vi "potentialField.vi"(5 "Ball":refnum<class "Ball.lvclass">, 7 "enemyRobots":refnum<class "Robot.lvclass">[](array[class]), 8 "error in (no error)":errorcluster, 11 "Robot in":refnum<class "Robot.lvclass">) -> (0 "error out":errorcluster, 3 "Robot out":refnum<class "Robot.lvclass">)   [LabVIEW 2020, in "Robot.lvclass"]
uses:
  Robot.lvclass
  C:/RoboIME/SSL_AI/Object_class/Object.lvclass
  Ball_class/Ball.lvclass
  <vilib>/Analysis/_algsub.llb/Vector Norm Type.ctl
  Robot.lvclass/Robot.ctl
  Object_class/Object.lvclass/Object.ctl
  obstacle.ctl
  Object_class/Read x.vi
  Object_class/Read y.vi
  <vilib>/Analysis/_algsub.llb/Real Vector Norm.vi
  Object_class/Read position(x,y).vi
  <vilib>/Analysis/coordinate.llb/2D Cartesian Coordinate Rotation (Scalar).vi
  Read robotKickState.vi
  Read dest_x.vi
  Read dest_y.vi
  Read v_tang.vi
  Read v_norm.vi
  Read orientation.vi
  Write v_tang.vi
  Write v_norm.vi
  <vilib>/Analysis/NI_AALPro.lvlib
panel:
  in  "multiplier(ball)":dbl(slide)=0.5102040816326531 scale=0.0..10.0
  in  "influence radius(ball)":dbl=400.0 format="%#_13g"
  in  "multiplier(enemy)":dbl(slide)=2.9591836734693877 scale=0.0..10.0
  in  "influence radius(enemy)":dbl=600.0 format="%#_13g"
  in  "min dist to reduce":dbl=500.0 format="%#_13g"
  in  "dist to nullify pot field":dbl=800.0 format="%#_13g"
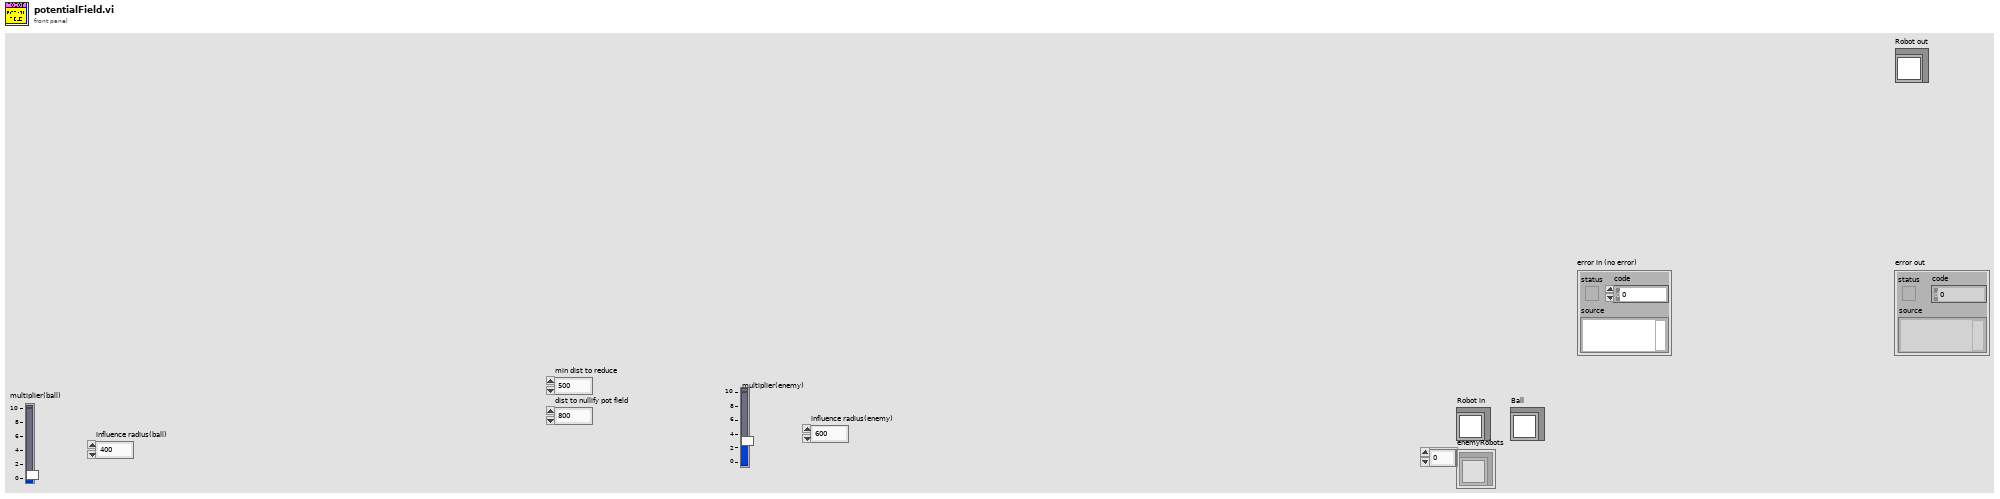
[diagram p1: front panel]
types:
  T1 = typedef "NI_AALPro.lvlib/Vector Norm Type.ctl" = u16
  T2 = typedef "robotKickToStates.ctl" = enum16{"stop", "oldKickTo", "shootFromDirect", "avoidCollideBall", "goToBackBall", "none", "walk", "turn", "oldKickToShoot", "oldKickToGoToBackBall", "shoot"}
  T3 = typedef "obstacle.ctl" = cluster{"x":dbl, "y":dbl, "influenceRadius":dbl, "multiplier":dbl}
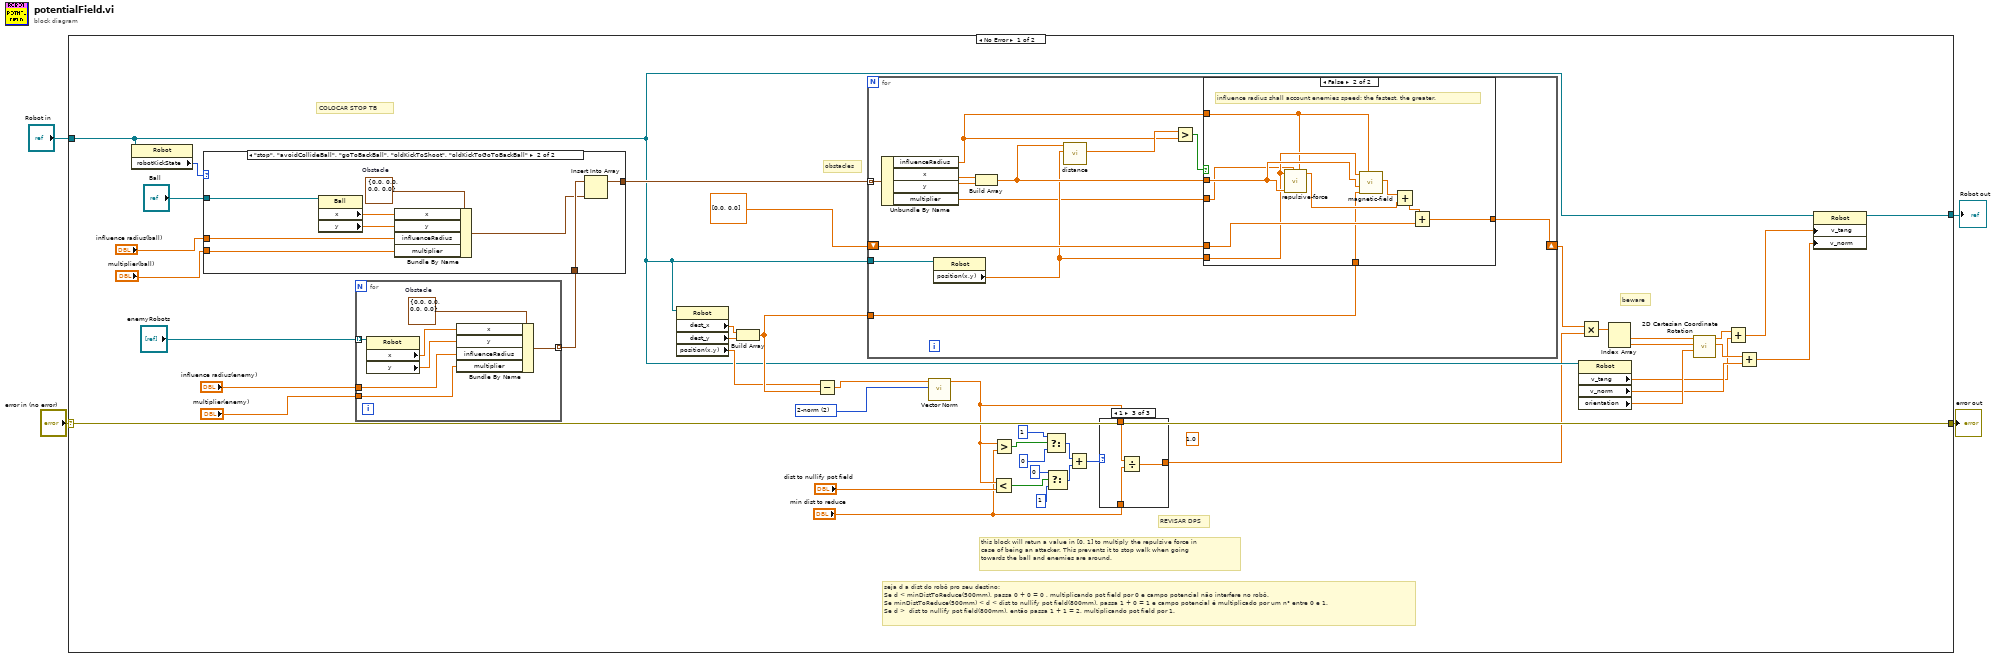
[diagram p0: block diagram]
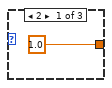
[diagram p2: hidden frame]
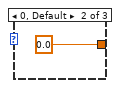
[diagram p3: hidden frame]
diagram:
  n1 = case shown="No Error" "error in (no error)" {
    selector: "error in (no error)" -> [w47 w95]
    tunnel: [w47 w95] -> w3
    tunnel: [w44 w94] -> w2
    tunnel: "Robot in" -> [w11 w94]
    frame No Error {
      (unwired) 1.0
      w36 = T1 2 items=["1-norm"=1, "2-norm"=2, "Inf-norm"=3, "-Inf-norm"=4, "User Defined"=5] ("norm type")
      # "COLOCAR STOP TB"
      # "seja d a dist do robô pro seu destino:\nSe d < minDistToReduce(500mm), passa 0 + 0 = 0 , multiplicando pot field por 0 e campo potencial não interfere no robô.\nSe minDistToReduce(500mm) < d < dist to nullify pot field(800mm), passa 1 + 0 = 1 e campo potencial é multiplicado por um n° entre 0 e 1.\nSe d >  dist to nullify pot field(800mm), então passa 1 + 1 = 2, multiplicando pot field por 1."
      # "REVISAR DPS"
      # "obstacles"
      # "this block will retun a value in [0, 1] to multiply the repulsive force in\ncase of being an attacker. This prevents it to stop walk when going \ntowards the ball and enemies are around."
      # "beware"
      n2 = property class="Robot"(reference=w11) -> ("robotKickState"=w10:T2)  [unwired: 1 in, 2 out]
      n3 = for {
        tunnel: "enemyRobots" -> [w93] mode=indexing
        tunnel: [w90] -> w43 mode=indexing
        tunnel: "influence radius(enemy)" -> [w88]
        tunnel: "multiplier(enemy)" -> [w87]
        w89 = T3 {"x"=0.0, "y"=0.0, "influenceRadius"=0.0, "multiplier"=0.0}  # Obstacle
        n4 = property class="Robot"(reference=w93) -> ("x"=w92:dbl, "y"=w91:dbl)  [unwired: 1 in, 2 out]
        n5 = Bundle By Name(cluster=w89, "x"=w92, "y"=w91, "influenceRadius"=w88, "multiplier"=w87) -> (w90:T3)
      }
      n6 = case shown="\"stop\", \"avoidCollideBall\", \"goToBackBall\", \"oldKickToShoot\", \"oldKickToGoToBackBall\"" w10 {
        tunnel: "Ball" -> [_ w86]
        tunnel: w43 -> [w77 w82]
        tunnel: [w77 w80] -> w42
        tunnel: "influence radius(ball)" -> [_ w79]
        tunnel: "multiplier(ball)" -> [_ w78]
        frame Default {
        }
        frame "stop", "avoidCollideBall", "goToBackBall", "oldKickToShoot", "oldKickToGoToBackBall" {
          w85 = T3 {"x"=0.0, "y"=0.0, "influenceRadius"=0.0, "multiplier"=0.0}  # Obstacle
          n7 = property class="Ball"(reference=w86) -> ("x"=w84:dbl, "y"=w83:dbl)  [unwired: 1 in, 2 out]
          n8 = Bundle By Name(cluster=w85, "x"=w84, "y"=w83, "influenceRadius"=w79, "multiplier"=w78) -> (w81:T3)
          n9 = Insert Into Array(array=w82, new element=w81) -> (w80:T3[])  [unwired: 1 in]
        }
      }
      n10 = property class="Robot"(reference=w11) -> ("dest_x"=w19:dbl, "dest_y"=w18:dbl, "position(x,y)"=w20:dbl[])  [unwired: 1 in, 2 out]
      n11 = Build Array(w19, w18) -> (w34:dbl[])
      n12 = Subtract(x=w20, y=w34) -> (x-y=w37:dbl[])
      n13 = for {
        tunnel: w42 -> [w65] mode=indexing
        tunnel: w11 -> [w56]
        shift-right: [w61] -> w39
        shift-left: dbl[] [0.0, 0.0] -> [w62]
        tunnel: w34 -> [w59]
        n14 = Unbundle By Name(w65) -> ("influenceRadius"=w54:dbl, "x"=w64:dbl, "y"=w63:dbl, "multiplier"=w53:dbl)
        n15 = property class="Robot"(reference=w56) -> ("position(x,y)"=w55:dbl[])  [unwired: 1 in, 2 out]
        n16 = Build Array(w64, w63) -> (w60:dbl[])
        n17 = call "distance.vi"("P1"=w55, "P2"=w60) -> ("Dist P1P2"=w58:dbl)  [unwired: 9 in]
        n18 = Greater?(x=w58, y=w54) -> (0:w57:bool)
        n19 = case shown="False" w57 {
          tunnel: w62 -> [w66 w76]
          tunnel: [w66 w75] -> w61
          tunnel: w60 -> [_ w71]
          tunnel: w55 -> [_ w70]
          tunnel: w59 -> [_ w69]
          tunnel: w54 -> [_ w68]
          tunnel: w53 -> [_ w67]
          frame True {
          }
          frame False {
            # "influence radius shall account enemies speed: the fastest, the greater."
            n20 = call "repulsive-force.vi"("influence radius"=w68, "multiplier"=w67, "obstacle pos"=w71, "agent pos"=w70) -> ("force"=w73:dbl[])  [unwired: 6 in, 1 out]
            n21 = call "magnetic-field.vi"("obstacle influence radius"=w68, "goal pos"=w69, "obstacle pos"=w71, "ally pos"=w70) -> ("magnetic force"=w74:dbl[])  [unwired: 7 in]
            n22 = Add(x=w74, y=w73) -> (x+y=w72:dbl[])
            n23 = Add(x=w72, y=w76) -> (x+y=w75:dbl[])
          }
        }
      }
      n24 = call-poly <vilib>:"Vector Norm.vi"("norm type"=w36, "Input Vector"=w37) -> ("norm"=w35:dbl)  [unwired: 8 in, 1 out]
      n25 = Less?(x=w35, y="dist to nullify pot field") -> (x < y?=w30:bool)
      n26 = Greater?(x=w35, y="min dist to reduce") -> (0:w31:bool)
      n27 = Select(t=1, s=w31, f=0) -> (s? t:f=w32:i32)
      n28 = Select(t=0, s=w30, f=1) -> (s? t:f=w33:i32)
      n29 = Add(x=w32, y=w33) -> (x+y=w24:i32)
      n30 = case shown="1" w24 {
        tunnel: [1.0 0.0 w50] -> w9
        tunnel: w35 -> [_ _ w52]
        tunnel: "min dist to reduce" -> [_ _ w51]
        frame 2 {
        }
        frame 0, Default {
        }
        frame 1 {
          n31 = Divide(x=w52, y=w51) -> (x/y=w50:dbl)
        }
      }
      n32 = property class="Robot"(reference=w11) -> ("v_tang"=w12:dbl, "v_norm"=w14:dbl, "orientation"=w17:dbl)  [unwired: 1 in, 2 out]
      n33 = Multiply(x=w39, y=w9) -> (x*y=w38:dbl[])
      n34 = Index Array(array=w38) -> (element #1=w16:dbl, element #2=w41:dbl)  [unwired: 2 in]
      n35 = call-poly <vilib>:"2D Cartesian Coordinate Rotation.vi"("theta"=w17, "y"=w41, "x"=w16) -> ("y out"=w15:dbl, "x out"=w13:dbl)  [unwired: 6 in, 1 out]
      n36 = Add(x=w13, y=w12) -> (x+y=w22:dbl)
      n37 = Add(x=w15, y=w14) -> (x+y=w21:dbl)
      n38 = property class="Robot"(reference=w11, "v_tang"=w22, "v_norm"=w21) -> (reference out=w44:refnum<class "Robot.lvclass">)  [unwired: 1 in, 1 out]
    }
    frame Error {
    }
  }
  "error out" <- w3
  "Robot out" <- w2
